vi "RT Loop - Watchdog.vi"(11 "Message Queue":refnum<queue> caption="消息队列") -> ()   [LabVIEW 2013]
uses:
  support/Message Queue/Message Cluster.ctl
  <vilib>/RTwatchdog.llb/Watchdog expiration actions.ctl
  <vilib>/RTwatchdog.llb/Watchdog status enum.ctl
  Globals/Global - Configuration Options.vi
  Globals/Global - All RT Loop Stop.vi
  support/Message Queue/Message Queue.lvlib
panel:
  in  "expiration actions":T1={"reset"=TRUE, "occurrence"=FALSE, "trigger protocol"=enum."active high", "trigger line"=enum."none", "disable watchdog on VI exit"=TRUE}
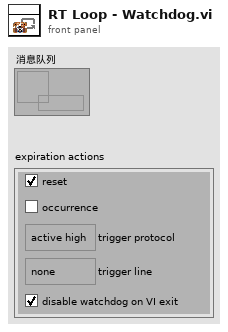
[diagram p1: front panel]
types:
  T1 = typedef "Watchdog expiration actions.ctl" = cluster{"reset":bool, "occurrence":bool, "trigger protocol":enum16{"active high", "active low", "open collector"}, "trigger line":enum16{"none", "line 0", "line 1", "line 2", "line 3", "line 4", "line 5", "line 6", "line 7", "SMB line 0"}, "disable watchdog on VI exit":bool}
  T2 = typedef "Watchdog status enum.ctl" = enum16{"disabled", "expired", "running"}
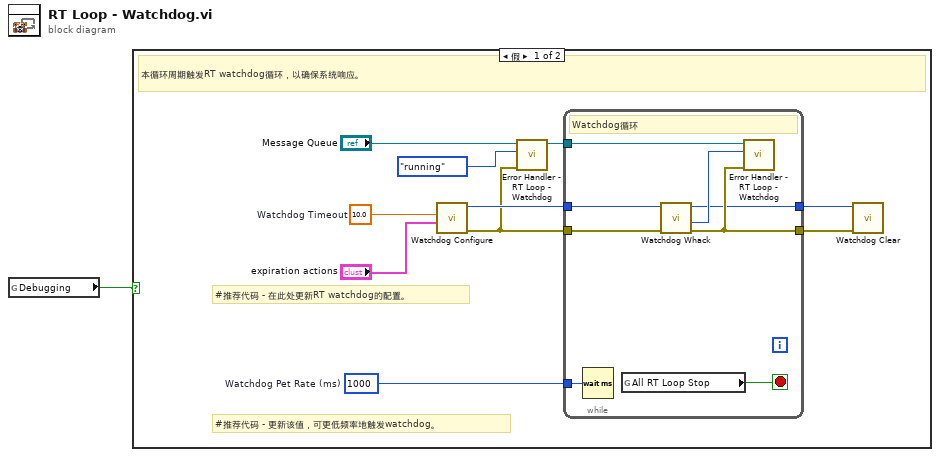
[diagram p0: block diagram]
diagram:
  n1 = global read "Global - Configuration Options.vi" "Debugging"() -> (w1:bool)
  n2 = case shown="假" w1 {
    frame False {
      w7 = u32 1000  # Watchdog Pet Rate (ms)
      w9 = 10.0  # Watchdog Timeout
      # "#推荐代码 - 在此处更新RT watchdog的配置。"
      # "#推荐代码 - 更新该值，可更低频率地触发watchdog。"
      # "本循环周期触发RT watchdog循环，以确保系统响应。"
      n3 = call <vilib>:"Watchdog Configure.vi"("expiration actions"="expiration actions", "timeout (1 sec)"=w9) -> ("error out"=w4:errorcluster, "watchdogID"=w10:u32)  [unwired: 2 in, 2 out]
      n4 = call "Error Handler - RT Loop - Watchdog.vi"("error in (no error)"=w4, "watchdog status"=Watchdog_status_enum."running", "Message Queue"="Message Queue") -> ("dup Message Queue"=w11:refnum<queue>)  [unwired: 8 in]
      n5 = while {
        tunnel: w11 -> [w18]
        tunnel: w10 -> [w16]
        tunnel: w7 -> [w17]
        tunnel: [w12] -> w2
        tunnel: w4 -> [w14]
        tunnel: [w13] -> w3
        stop <- w19 stop-if-true
        # "Watchdog循环"
        n6 = Wait (ms)(milliseconds to wait=w17) -> ()  [unwired: 1 out]
        n7 = global read "Global - All RT Loop Stop.vi" "All RT Loop Stop"() -> (w19:bool)
        n8 = call <vilib>:"Watchdog Whack.vi"("error in (no error)"=w14, "watchdogID in"=w16) -> ("error out"=w13:errorcluster, "watchdog status"=w15:T2, "watchdogID out"=w12:u32)  [unwired: 3 in]
        n9 = call "Error Handler - RT Loop - Watchdog.vi"("error in (no error)"=w13, "watchdog status"=w15, "Message Queue"=w18) -> ()  [unwired: 8 in, 1 out]
      }
      n10 = call <vilib>:"Watchdog Clear.vi"("error in (no error)"=w3, "watchdogID in"=w2) -> ()  [unwired: 5 in, 1 out]
    }
    frame True {
      # "调试时不能启用watchdog。"
    }
  }
